vi "init.vi"(0 "VrefTest in":refnum<class "VrefTest.lvclass">, 1 "Tolerance":dbl[unit], 5 "Log":refnum<class "ITestLog.lvclass">, 7 "DAQ Channel To Read":refnum<k21>, 9 "Expected Value":dbl[unit], 11 "error in (no error)":errorcluster, 12 "Samples To Read":dbl) -> (4 "VrefTest out":refnum<class "VrefTest.lvclass">, 15 "error out":errorcluster)   [LabVIEW 2015, in "VrefTest.lvclass"]
uses:
  VrefTest.lvclass
  Model/TestLog/ITestLog/ITestLog.lvclass
  VrefTest.lvclass/VrefTest.ctl
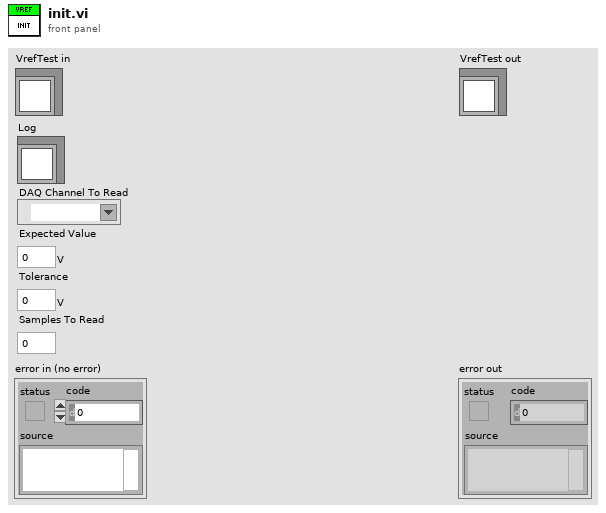
[diagram p1: front panel]
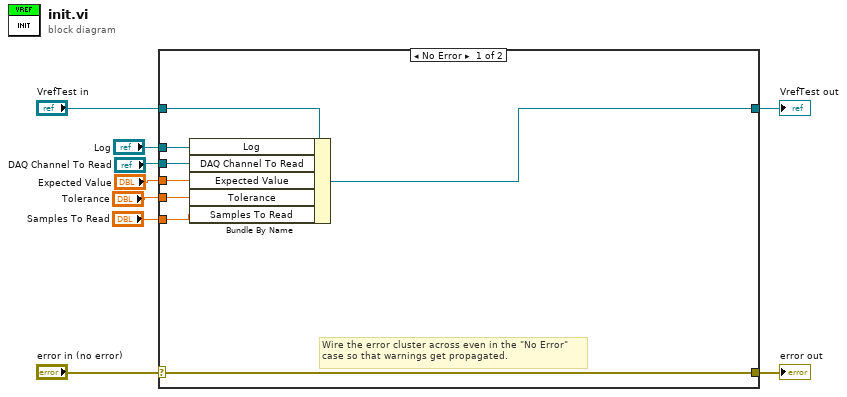
[diagram p0: block diagram]
diagram:
  n1 = case shown="No Error" "error in (no error)" {
    selector: "error in (no error)" -> [w17 w19]
    tunnel: [w17 w19] -> w8
    tunnel: [w10 w18] -> w6
    tunnel: "VrefTest in" -> [w11 w18]
    tunnel: "Log" -> [w14 _]
    tunnel: "DAQ Channel To Read" -> [w16 _]
    tunnel: "Expected Value" -> [w15 _]
    tunnel: "Tolerance" -> [w13 _]
    tunnel: "Samples To Read" -> [w12 _]
    frame No Error {
      # "Wire the error cluster across even in the \"No Error\"\ncase so that warnings get propagated."
      n2 = Bundle By Name(cluster=w11, "Log"=w14, "DAQ Channel To Read"=w16, "Expected Value"=w15, "Tolerance"=w13, "Samples To Read"=w12) -> (w10:refnum<class "VrefTest.lvclass">)
    }
    frame Error {
    }
  }
  "error out" <- w8
  "VrefTest out" <- w6
